vi "readInLimitsFromXML.vi"(6 "type":string, 8 "error in (no error)":errorcluster, 9 "device.lvclass":refnum<class "device.lvclass">, 10 "xml in":refnum<class "NativeXML.lvclass">, 11 "deviceDataBase in":refnum<class "deviceDataBase.lvclass">) -> (0 "error out":errorcluster, 1 "device.lvclass out":refnum<class "device.lvclass">, 2 "xml out":refnum<class "NativeXML.lvclass">, 3 "deviceDataBase out":refnum<class "deviceDataBase.lvclass">)   [LabVIEW 2011, in "Tools.lvlib" / "DatabaseHelpers.lvlib" / "deviceDataBase.lvclass"]
uses:
  deviceDataBase.lvclass
  Database Objects/device/device.lvclass
  NativeXML/NativeXML.lvclass
  Database Objects/device/AnalogDevice/AnalogDevice.lvclass
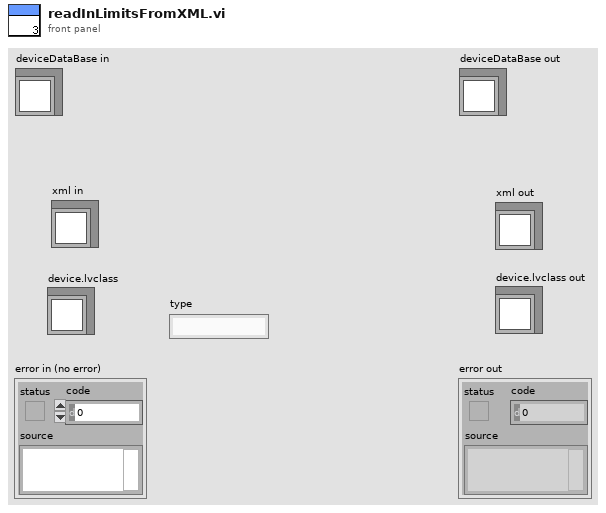
[diagram p1: front panel]
types:
  T1 = cluster{"VoltageLimit":dbl, "CurrentLimit":dbl}[]
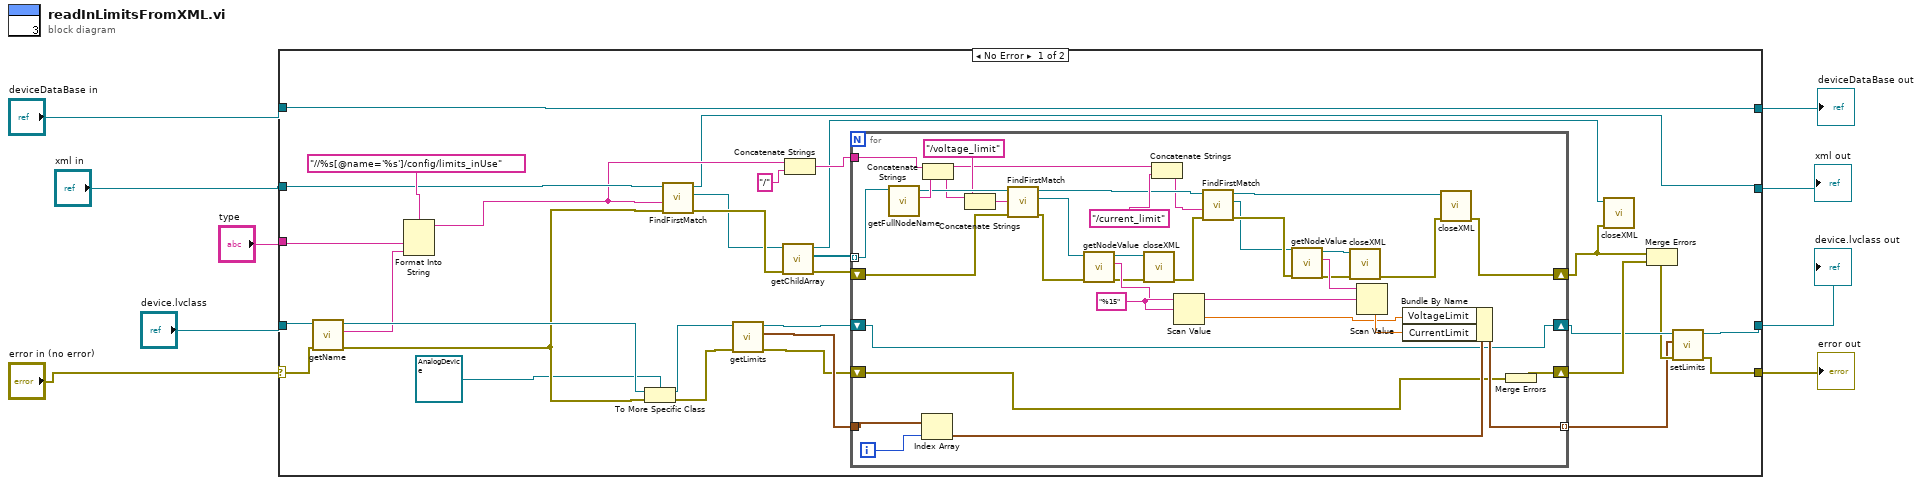
[diagram p0: block diagram]
diagram:
  n1 = case shown="No Error" "error in (no error)" {
    selector: "error in (no error)" -> [w34 w79]
    tunnel: [w11 w79] -> w1
    tunnel: [w40 w78] -> w4
    tunnel: "xml in" -> [w26 w77]
    tunnel: "device.lvclass" -> [w36 w76]
    tunnel: [w14 w76] -> w2
    tunnel: [w23 w77] -> w3
    tunnel: "deviceDataBase in" -> [w40 w78]
    tunnel: "type" -> [w33 _]
    frame No Error {
      n2 = call "getName.vi"("error in (no error)"=w34, "device.lvclass in"=w36) -> ("error out"=w25:errorcluster, "name"=w32:string, "device.lvclass out"=w35:refnum<class "device.lvclass">)  [unwired: 7 in]
      n3 = Format Into String(format string="//%s[@name='%s']/config/limits_inUse", w33, w32) -> (resulting string=w24:string)  [unwired: 2 in, 1 out]
      n4 = To More Specific Class(target class=refnum<class "AnalogDevice.lvclass"> refnum ("Tools.lvlib:DatabaseHelpers.lvlib:AnalogDevice.lvclass"), reference=w35, error in=w25) -> (specific class reference=w15:refnum<class "AnalogDevice.lvclass">, error out=w16:errorcluster)
      n5 = call "FindFirstMatch.vi"("error in (no error)"=w25, "xPath"=w24, "NativeXML in"=w26) -> ("error out"=w22:errorcluster, "NativeXML match"=w21:refnum<class "NativeXML.lvclass">, "NativeXML out"=w23:refnum<class "NativeXML.lvclass">)  [unwired: 6 in]
      n6 = call "getLimits.vi"("error in (no error)"=w16, "AnalogDevice in"=w15) -> ("error out"=w17:errorcluster, "Limits"=w18:T1, "AnalogDevice out"=w19:refnum<class "AnalogDevice.lvclass">)  [unwired: 7 in]
      n7 = call "getChildArray.vi"("error in (no error)"=w22, "NativeXML in"=w21) -> ("error out"=w38:errorcluster, "childArray"=w39:refnum<class "NativeXML.lvclass">[], "NativeXML out"=w27:refnum<class "NativeXML.lvclass">)  [unwired: 7 in]
      n8 = Concatenate Strings(w24, "/") -> (w29:string)
      n9 = for {
        shift-right: [w70] -> w13
        shift-left: w19 -> [w70]
        shift-right: [w74] -> w37
        shift-left: w17 -> [w69]
        tunnel: w39 -> [w61] mode=indexing
        tunnel: w18 -> [w73]
        tunnel: [w75] -> w10 mode=indexing
        shift-right: [w55] -> w28
        shift-left: w38 -> [w53]
        tunnel: w29 -> [w62]
        i -> [w71]
        w68 = "%15"
        n10 = call "getFullNodeName.vi"("NativeXML in"=w61) -> ("fullName"=w63:string, "NativeXML out"=w54:refnum<class "NativeXML.lvclass">)  [unwired: 8 in, 1 out]
        n11 = Index Array(array=w73, index=w71) -> (element=w72:cluster{"VoltageLimit":dbl, "CurrentLimit":dbl})
        n12 = Concatenate Strings(w62, w63) -> (w48:string)
        n13 = Concatenate Strings(w48, "/voltage_limit") -> (w49:string)
        n14 = call "FindFirstMatch.vi"("error in (no error)"=w53, "xPath"=w49, "NativeXML in"=w54) -> ("error out"=w52:errorcluster, "NativeXML match"=w51:refnum<class "NativeXML.lvclass">, "NativeXML out"=w45:refnum<class "NativeXML.lvclass">)  [unwired: 6 in]
        n15 = call "getNodeValue.vi"("error in (no error)"=w52, "NativeXML in"=w51) -> ("error out"=w59:errorcluster, "Value"=w65:string, "NativeXML out"=w60:refnum<class "NativeXML.lvclass">)  [unwired: 7 in]
        n16 = call "closeXML.vi"("error in (no error)"=w59, "NativeXML in"=w60) -> ("error out"=w43:errorcluster)  [unwired: 9 in]
        n17 = Concatenate Strings(w48, "/current_limit") -> (w44:string)
        n18 = Scan Value(string=w65, format string=w68) -> (value=w66:dbl)  [unwired: 1 in, 1 out]
        n19 = call "FindFirstMatch.vi"("error in (no error)"=w43, "xPath"=w44, "NativeXML in"=w45) -> ("error out"=w42:errorcluster, "NativeXML match"=w41:refnum<class "NativeXML.lvclass">, "NativeXML out"=w46:refnum<class "NativeXML.lvclass">)  [unwired: 6 in]
        n20 = call "getNodeValue.vi"("error in (no error)"=w42, "NativeXML in"=w41) -> ("error out"=w58:errorcluster, "Value"=w64:string, "NativeXML out"=w57:refnum<class "NativeXML.lvclass">)  [unwired: 7 in]
        n21 = call "closeXML.vi"("error in (no error)"=w58, "NativeXML in"=w57) -> ("error out"=w56:errorcluster)  [unwired: 9 in]
        n22 = Scan Value(string=w64, format string=w68) -> (value=w67:dbl)  [unwired: 1 in, 1 out]
        n23 = Bundle By Name(cluster=w72, "VoltageLimit"=w66, "CurrentLimit"=w67) -> (w75:cluster{"VoltageLimit":dbl, "CurrentLimit":dbl})
        n24 = call "closeXML.vi"("error in (no error)"=w56, "NativeXML in"=w46) -> ("error out"=w55:errorcluster)  [unwired: 9 in]
        n25 = Merge Errors(w69) -> (w74:errorcluster)
      }
      n26 = call "closeXML.vi"("error in (no error)"=w28, "NativeXML in"=w27) -> ()  [unwired: 9 in, 1 out]
      n27 = Merge Errors(w28, w37) -> (w12:errorcluster)
      n28 = call "setLimits.vi"("error in (no error)"=w12, "Limits"=w10, "AnalogDevice in"=w13) -> ("error out"=w11:errorcluster, "AnalogDevice out"=w14:refnum<class "AnalogDevice.lvclass">)  [unwired: 7 in]
    }
    frame Error {
    }
  }
  "error out" <- w1
  "deviceDataBase out" <- w4
  "xml out" <- w3
  "device.lvclass out" <- w2
